vi "GetDPIValuesFromMode.vi"(11 "PrintMode":string="360dpi x 360dpi (1dpd) CMYK+Blue+Orange") -> (0 "Y_res":i32, 1 "X_res":i32, 2 "y":i32, 3 "x":i32)   [LabVIEW 2022 SP3]
uses:
  <vilib>/regexp/Match Regular Expression.xnode
panel:
  out "Array":string[](array[string])
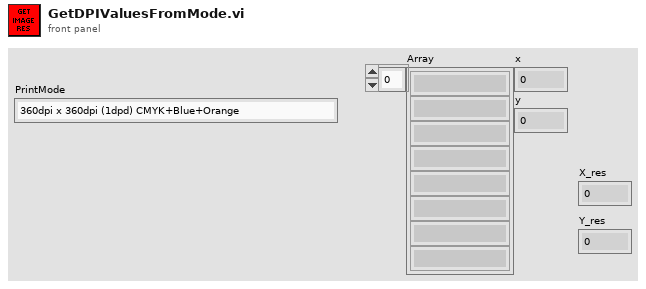
[diagram p1: front panel]
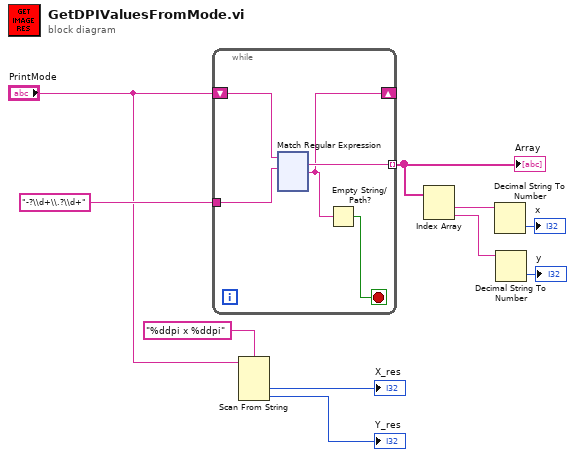
[diagram p0: block diagram]
diagram:
  n1 = while {
    tunnel: "-?\\d+\\.?\\d+" -> [w14]
    shift-right: [w12] -> _
    shift-left: "PrintMode" -> [w15]
    tunnel: [w13] -> w9 mode=indexing
    stop <- w11 stop-if-true
    n2 = xnode "Match Regular Expression"("input string"=w15, "regular expression"=w14) -> ("whole match"=w13:string, "after match"=w12:string)  [unwired: 4 in, 3 out]
    n3 = Empty String/Path?(string/path=w12) -> (empty?=w11:bool)
  }
  "Array" <- w9
  n4 = Scan From String(format string="%ddpi x %ddpi", input string="PrintMode") -> (output 1=→"X_res":i32, output 2=→"Y_res":i32)  [unwired: 4 in, 3 out]
  n5 = Index Array(array=w9) -> (element #1=w8:string, element #2=w7:string)  [unwired: 2 in]
  n6 = Decimal String To Number(string=w8) -> (number=→"x":i32)  [unwired: 2 in, 1 out]
  n7 = Decimal String To Number(string=w7) -> (number=→"y":i32)  [unwired: 2 in, 1 out]
